vi "Thermistor_Arduino_ContSample.vi"() -> ()   [LabVIEW 2018]
uses:
  <vilib>/express/express shared/transition.llb/Dynamic To Waveform Array.vi
  <vilib>/express/express arith-compare/Formula/Block/exnFormulaBlock how many pts in the wave.vi
  <vilib>/express/express shared/ex_Modify Signal Name.vi
  <vilib>/express/express shared/transition.llb/Waveform Array To Dynamic.vi
  <vilib>/express/express arith-compare/Formula/XNode/ExpressFormulaBlockNode.xnode
  <vilib>/LabVIEW Interface for Arduino/LabVIEW Interface for Arduino.lvlib
panel:
  out "Numeric":dbl
  in  "Sample Rate":u16
  in  "Analog Input Pin":u8
  out "Temperature Chart":dynamicdata(graph)
  out "Temperature (Celcius)":dbl(slide) scale=0.0..100.0
  in  "Set Voltage \nFor Simulation":dbl(knob) scale=0.0..5.0
  out "Temperature (Kelvin)":dbl
  in  "Stop The System":bool
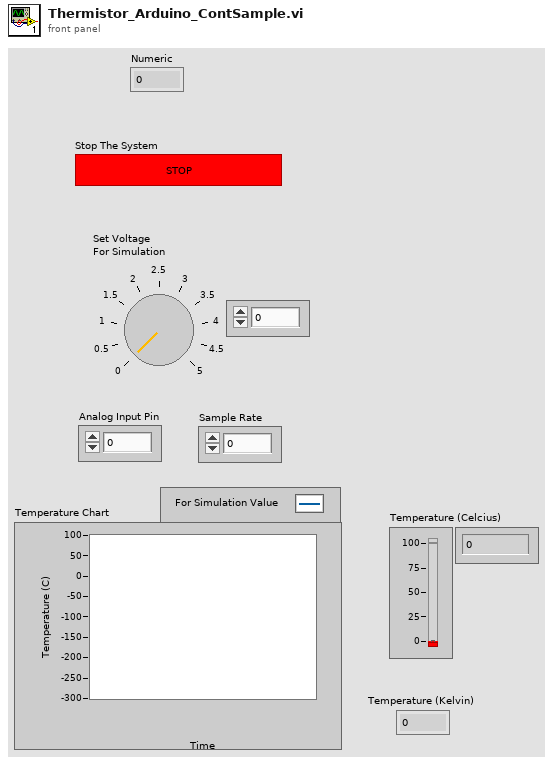
[diagram p1: front panel]
types:
  T1 = typedef "LabVIEW Interface for Arduino.lvlib/Arduino Resource.ctl" = cluster{"VISA resource":refnum<visa-resource-name>, "Board Type":T2, "Connection Type":enum8{"USB / Serial"}, "Bytes Per Packet (15)":u8}
  T2 = typedef "LabVIEW Interface for Arduino.lvlib/Board Type.ctl" = enum16{"Uno", "Dimuelanove w/Atmega 328", "Mega 2560"}
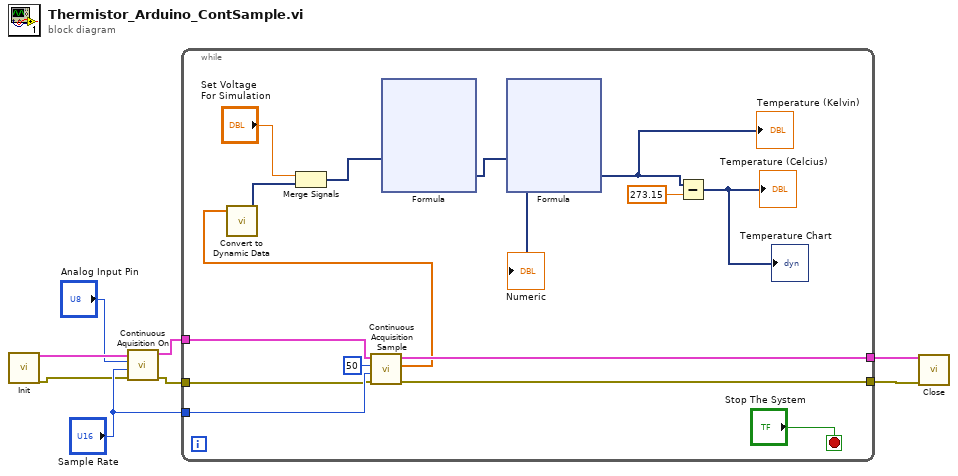
[diagram p0: block diagram]
diagram:
  n1 = call <vilib>:"Init.vi"() -> ("Arduino Resource"=w4:T1, "error out"=w5:errorcluster)  [unwired: 18 in]
  n2 = call <vilib>:"Continuous Aquisition On.vi"("error in"=w5, "Acquition Speed"="Sample Rate", "Analog Input Pin"="Analog Input Pin", "Arduino Resource"=w4) -> ("error out"=w3:errorcluster, "Arduino Resource"=w2:T1)  [unwired: 6 in]
  n3 = while {
    tunnel: [w23] -> w8
    tunnel: [w22] -> w7
    tunnel: "Sample Rate" -> [w14]
    tunnel: w3 -> [w13]
    tunnel: w2 -> [w12]
    stop <- "Stop The System" stop-if-true
    n4 = call <vilib>:"Continuous Acquisition Sample.vi"("Arduino Resource"=w12, "Samples to Read"=u16 50, "Sample Rate (HZ)"=w14, "error in (no error)"=w13) -> ("Arduino Resource"=w23:T1, "Data"=w15:dbl[], "error out"=w22:errorcluster)  [unwired: 4 in]
    n5 = call "Convert to Dynamic Data"("Array"=w15) -> ("Dynamic Data Type"=w9:dynamicdata)  [unwired: 3 in]
    n6 = Merge Signals("Set Voltage \nFor Simulation", w9) -> (w11:dynamicdata)
    n7 = xnode "Formula"("X1"=w11) -> ("Result"=w21:dynamicdata)  [unwired: 1 in, 1 out]
    "Numeric" <- w21
    n8 = xnode "Formula"("X1"=w21) -> ("Result"=w18:dynamicdata)  [unwired: 1 in, 1 out]
    "Temperature (Kelvin)" <- w18
    n9 = Subtract(x=w18, y=273.15) -> (x-y=→"Temperature (Celcius)" →"Temperature Chart":dynamicdata)
  }
  n10 = call <vilib>:"Close.vi"("Arduino Resource"=w8, "error in"=w7) -> ()  [unwired: 13 in, 1 out]
